vi "Set Values From HovaCAL Output.vi"(8 "error in (no error)":errorcluster caption="Fehler (Eingang, kein Fehler)") -> (0 "error out":errorcluster caption="Fehler (Ausgang)", 1 "Cluster.Flow Output Cluster (Ausgang)":cluster{"total flow":dbl} caption="Flow Output", 2 "Cluster.Pump MassFlow-Cluster":T7(array[cluster]) caption="Pump MassFlow", 3 "Cluster.Pump Concentrations-Cluster":T8(array[cluster]) caption="Pump Output", 4 "Cluster.PumpModeGeneral-Cluster":cluster{"running?":bool, "Speed":dbl[]} caption="Pump Status", 5 "Cluster.Temp Cluster":T1(array[cluster]) caption="Temp Output", 6 "Cluster.MFC Flows-Cluster":T6(array[cluster]), 7 "MFC Input/Output Concentrations (Ausgang)":T9[](array[typedef]) caption="MFC Input/Output" {"Input Concentration" format="%.2f"; "Output Setpoint" format="%.2f"; "flow expected" format="%.2f"; "flow actual" format="%.2f"; "output concentration dry" format="%.2f"; "output concentration" format="%.2f"}, 9 "Water-Cluster out":cluster{"water conc SP":dbl, "water conc":dbl}, 10 "PumpMode-Cluster":T4(array[cluster]) {"concentratio mode" items=["water", "reagent"]; "Reagent" items=["HCl", "HF", "NH3", "HG", "PPM", "ORGANIC"]}, 11 "MFC Output Array":T5[](array[typedef]) {"flow expected" format="%.2f"; "flow actual" format="%.2f"; "output concentration dry" format="%.2f"; "output concentration" format="%.2f"})   [LabVIEW 2020, in "Linearisierung v2.lvlib" / "Gasteiler.lvlib" / "HovaCAL_Interface.lvlib" / "Kommunikation.lvlib"]
uses:
  Kommunikation.lvlib
  Controls/MFC Output.ctl
  Controls/Pump Concentration Mode.ctl
  Controls/Reagent.ctl
  Aktion_FGV_HovaCAL_Interface_GetData.ctl
  Controls/Controls.lvlib
  Controls/MFC Output plus Input Output Concentrations.ctl
panel:
  # "l/min"
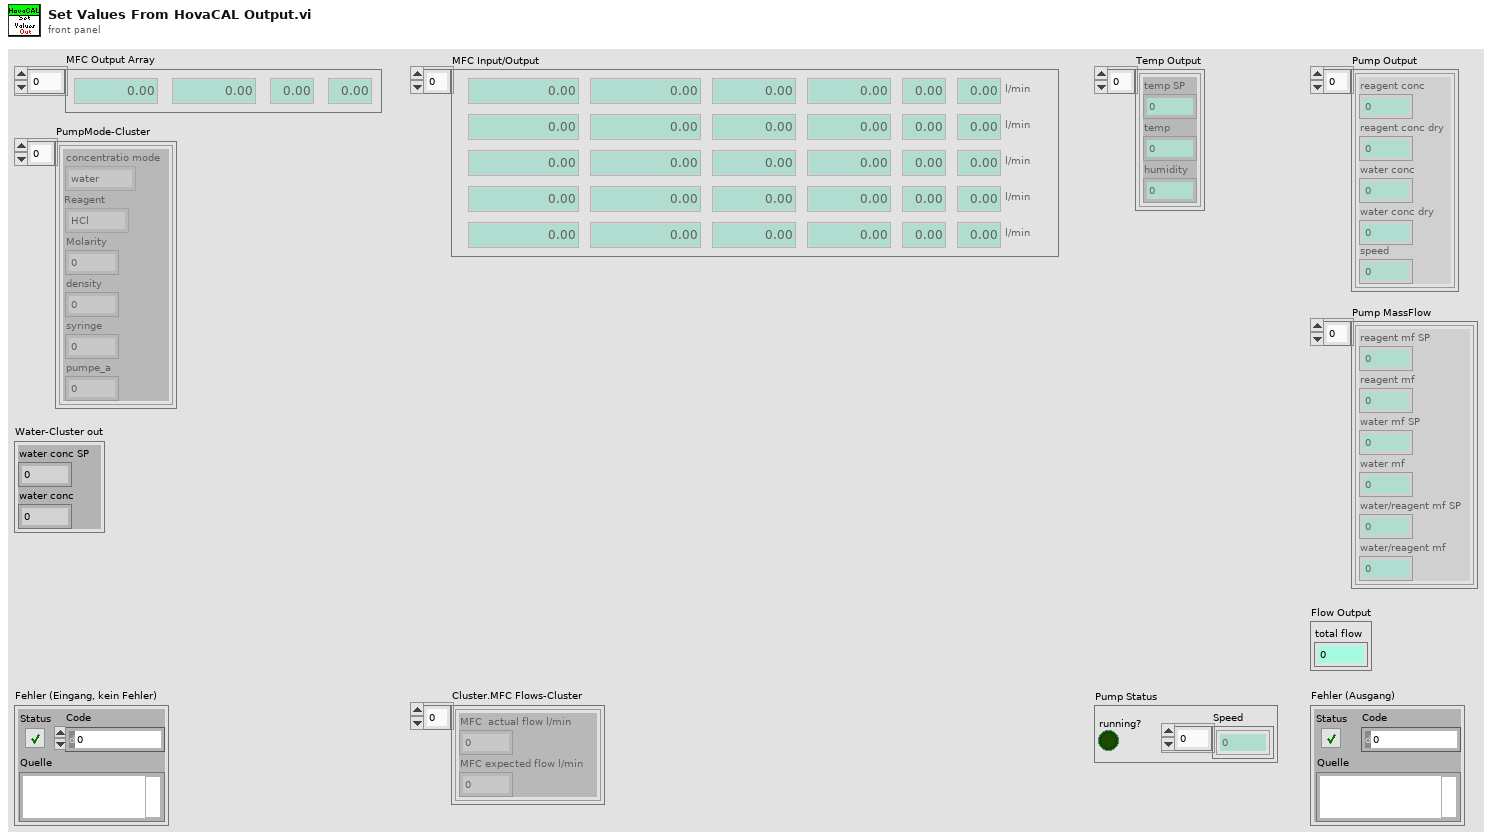
[diagram p1: front panel]
types:
  T1 = cluster{"temp SP":dbl, "temp":dbl, "humidity":dbl}[]
  T2 = typedef "Linearisierung v2.lvlib/Gasteiler.lvlib/HovaCAL_Interface.lvlib/Controls.lvlib/Pump Concentration Mode.ctl" = i32
  T3 = typedef "Linearisierung v2.lvlib/Gasteiler.lvlib/HovaCAL_Interface.lvlib/Controls.lvlib/Reagent.ctl" = i32
  T4 = cluster{"concentratio mode":T2, "Reagent":T3, "Molarity":dbl, "density":dbl, "syringe":dbl, "pumpe_a":dbl}[]
  T5 = typedef "Linearisierung v2.lvlib/Gasteiler.lvlib/HovaCAL_Interface.lvlib/Controls.lvlib/MFC Output.ctl" = cluster{"output concentration":dbl, "output concentration dry":dbl, "flow actual":dbl, "flow expected":dbl}
  T6 = cluster{"MFC  actual flow l/min":dbl, "MFC expected flow l/min":dbl}[]
  T7 = cluster{"reagent mf SP":dbl, "reagent mf":dbl, "water mf SP":dbl, "water mf":dbl, "water/reagent mf SP":dbl, "water/reagent mf":dbl}[]
  T8 = cluster{"reagent conc":dbl, "reagent conc dry":dbl, "water conc":dbl, "water conc dry":dbl, "speed":dbl}[]
  T9 = typedef "Linearisierung v2.lvlib/Gasteiler.lvlib/HovaCAL_Interface.lvlib/Controls.lvlib/MFC Output plus Input Output Concentrations.ctl" = cluster{"Input Concentration":dbl, "Output Setpoint":dbl, "output concentration":dbl, "output concentration dry":dbl, "flow actual":dbl, "flow expected":dbl}
  T10 = cluster{"temp SP":dbl, "temp":dbl, "humidity":dbl}
  T11 = cluster{"concentratio mode":T2, "Reagent":T3, "Molarity":dbl, "density":dbl, "syringe":dbl, "pumpe_a":dbl}
  T12 = cluster{"reagent conc":dbl, "reagent conc dry":dbl, "water conc":dbl, "water conc dry":dbl, "speed":dbl}
  T13 = typedef "Linearisierung v2.lvlib/Gasteiler.lvlib/HovaCAL_Interface.lvlib/Kommunikation.lvlib/Aktion_FGV_HovaCAL_Interface_GetData.ctl" = enum16{"lesen", "SystemInfo", "MFC Info", "actual Values", "Limits", "first contact", "reset after read"}
  T14 = typedef "Linearisierung v2.lvlib/Gasteiler.lvlib/HovaCAL_Interface.lvlib/Controls.lvlib/Pump Dry Mode.ctl" = i32
  T15 = typedef "Linearisierung v2.lvlib/Gasteiler.lvlib/HovaCAL_Interface.lvlib/Controls.lvlib/Pump Control Mode.ctl" = u32
  T16 = cluster{"Input Concentrations (Ausgang)":cluster{"input concentration setpoint":dbl, "output concentration setpoint":dbl, "output concentration":dbl, "output concentration dry":dbl}[], "Cluster":cluster{"Temp Cluster":cluster{"temp SP":dbl, "temp":dbl, "humidity":dbl}[], "PumpModeGeneral-Cluster":cluster{"running?":bool, "dry mode":T14, "control mode":T15}, "PumpMode-Cluster":cluster{"Speed":dbl, "concentratio mode":T2, "Reagent":T3, "Molarity":dbl, "density":dbl, "syringe":dbl, "pumpe_a":dbl}[], "Pump Concentrations-Cluster":cluster{"reagent conc SP":dbl, "reagent conc":dbl, "reagent conc dry":dbl, "water conc SP":dbl, "water conc":dbl, "water conc dry":dbl}[], "Flow Output Cluster (Ausgang)":cluster{"total flow setpoint":dbl, "total flow":dbl}, "Pump MassFlow-Cluster":cluster{"reagent mf SP":dbl, "reagent mf":dbl, "water mf SP":dbl, "water mf":dbl, "water/reagent mf SP":dbl, "water/reagent mf":dbl}[], "MFC Flows-Cluster":cluster{"MFC  actual flow l/min":dbl, "MFC expected flow l/min":dbl}[]}}
  T17 = cluster{"input concentration setpoint":dbl, "output concentration setpoint":dbl, "output concentration":dbl, "output concentration dry":dbl}[]
  T18 = cluster{"running?":bool, "dry mode":T14, "control mode":T15}
  T19 = cluster{"Speed":dbl, "concentratio mode":T2, "Reagent":T3, "Molarity":dbl, "density":dbl, "syringe":dbl, "pumpe_a":dbl}[]
  T20 = cluster{"reagent conc SP":dbl, "reagent conc":dbl, "reagent conc dry":dbl, "water conc SP":dbl, "water conc":dbl, "water conc dry":dbl}[]
  T21 = cluster{"total flow setpoint":dbl, "total flow":dbl}
  T22 = cluster{"reagent conc SP":dbl, "reagent conc":dbl, "reagent conc dry":dbl, "water conc SP":dbl, "water conc":dbl, "water conc dry":dbl}
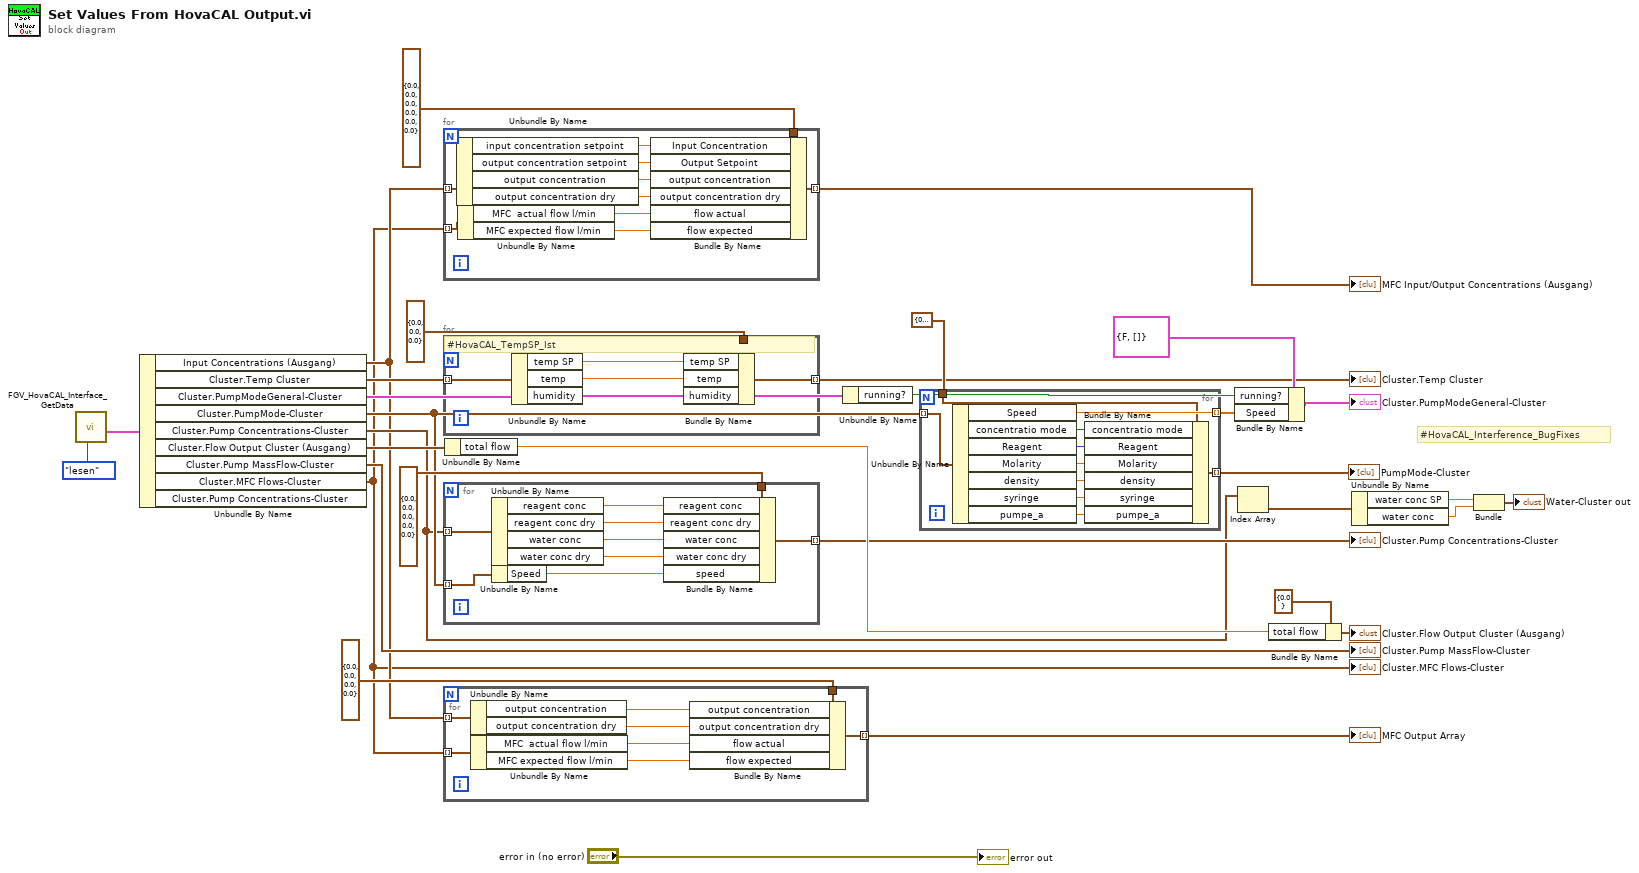
[diagram p0: block diagram]
diagram:
  # "#HovaCAL_Interference_BugFixes"
  n1 = call "FGV_HovaCAL_Interface_GetData.vi"("Aktion"=Aktion_FGV_HovaCAL_Interface_GetData."lesen") -> ("actual Values Cluster out"=w31:T16)  [unwired: 6 in, 4 out]
  n2 = Unbundle By Name(w31) -> ("Input Concentrations (Ausgang)"=w4:T17, "Cluster.Temp Cluster"=w30:T1, "Cluster.PumpModeGeneral-Cluster"=w28:T18, "Cluster.PumpMode-Cluster"=w9:T19, "Cluster.Pump Concentrations-Cluster"=w6:T20, "Cluster.Flow Output Cluster (Ausgang)"=w23:T21, "Cluster.Pump MassFlow-Cluster"=→"Cluster.Pump MassFlow-Cluster":T7, "Cluster.MFC Flows-Cluster"=w2:T6)  [unwired: 1 out]
  "Cluster.MFC Flows-Cluster" <- w2
  n3 = for {
    tunnel: w4 -> [w41] mode=indexing
    tunnel: T9 {"Input Concentration"=0.0, "Output Setpoint"=0.0, "output concentration"=0.0, "output concentration dry"=0.0, "flow actual"=0.0, "flow expected"=0.0} ("Actual Values Cluster") -> [w42]
    tunnel: [w39] -> w1 mode=indexing
    tunnel: w2 -> [w37] mode=indexing
    n4 = Unbundle By Name(w41) -> ("input concentration setpoint"=w33:dbl, "output concentration setpoint"=w34:dbl, "output concentration"=w40:dbl, "output concentration dry"=w38:dbl)
    n5 = Unbundle By Name(w37) -> ("MFC  actual flow l/min"=w35:dbl, "MFC expected flow l/min"=w36:dbl)
    n6 = Bundle By Name(cluster=w42, "Input Concentration"=w33, "Output Setpoint"=w34, "output concentration"=w40, "output concentration dry"=w38, "flow actual"=w35, "flow expected"=w36) -> (w39:T9)
  }
  "MFC Input/Output Concentrations (Ausgang)" <- w1
  n7 = for {
    tunnel: w30 -> [w48] mode=indexing
    tunnel: [w46] -> w13 mode=indexing
    tunnel: T10 {"temp SP"=0.0, "temp"=0.0, "humidity"=0.0} ("Temp Cluster") -> [w44]
    # "#HovaCAL_TempSP_Ist"
    n8 = Unbundle By Name(w48) -> ("temp SP"=w43:dbl, "temp"=w47:dbl, "humidity"=w45:dbl)
    n9 = Bundle By Name(cluster=w44, "temp SP"=w43, "temp"=w47, "humidity"=w45) -> (w46:T10)
  }
  "Cluster.Temp Cluster" <- w13
  n10 = for {
    tunnel: w6 -> [w56] mode=indexing
    tunnel: T12 {"reagent conc"=0.0, "reagent conc dry"=0.0, "water conc"=0.0, "water conc dry"=0.0, "speed"=0.0} ("Ausgangs-Cluster") -> [w57]
    tunnel: [w54] -> w11 mode=indexing
    tunnel: w9 -> [w50] mode=indexing
    n11 = Unbundle By Name(w56) -> ("reagent conc"=w55:dbl, "reagent conc dry"=w53:dbl, "water conc"=w52:dbl, "water conc dry"=w51:dbl)
    n12 = Unbundle By Name(w50) -> ("Speed"=w49:dbl)
    n13 = Bundle By Name(cluster=w57, "reagent conc"=w55, "reagent conc dry"=w53, "water conc"=w52, "water conc dry"=w51, "speed"=w49) -> (w54:T12)
  }
  "Cluster.Pump Concentrations-Cluster" <- w11
  n14 = for {
    tunnel: w2 -> [w64] mode=indexing
    tunnel: T5 {"output concentration"=0.0, "output concentration dry"=0.0, "flow actual"=0.0, "flow expected"=0.0} ("MFC Output") -> [w65]
    tunnel: [w63] -> w18 mode=indexing
    tunnel: w4 -> [w58] mode=indexing
    n15 = Unbundle By Name(w58) -> ("output concentration"=w60:dbl, "output concentration dry"=w59:dbl)
    n16 = Unbundle By Name(w64) -> ("MFC  actual flow l/min"=w62:dbl, "MFC expected flow l/min"=w61:dbl)
    n17 = Bundle By Name(cluster=w65, "output concentration"=w60, "output concentration dry"=w59, "flow actual"=w62, "flow expected"=w61) -> (w63:T5)
  }
  "MFC Output Array" <- w18
  n18 = Unbundle By Name(w23) -> ("total flow"=w21:dbl)
  n19 = Unbundle By Name(w28) -> ("running?"=w27:bool)
  n20 = for {
    tunnel: w9 -> [w75] mode=indexing
    tunnel: [w74] -> w25 mode=indexing
    tunnel: T11 {"concentratio mode"=0, "Reagent"=0, "Molarity"=0.0, "density"=0.0, "syringe"=0.0, "pumpe_a"=0.0} ("PumpMode-Cluster") -> [w73]
    tunnel: [w66] -> w12 mode=indexing
    n21 = Unbundle By Name(w75) -> ("Speed"=w74:dbl, "concentratio mode"=w72:T2, "Reagent"=w71:T3, "Molarity"=w70:dbl, "density"=w69:dbl, "syringe"=w68:dbl, "pumpe_a"=w67:dbl)
    n22 = Bundle By Name(cluster=w73, "concentratio mode"=w72, "Reagent"=w71, "Molarity"=w70, "density"=w69, "syringe"=w68, "pumpe_a"=w67) -> (w66:T11)
  }
  "PumpMode-Cluster" <- w12
  n23 = Bundle By Name(cluster=cluster{"running?":bool, "Speed":dbl[]} {"running?"=FALSE, "Speed"=[]} ("Cluster.PumpModeGeneral-Cluster"), "running?"=w27, "Speed"=w25) -> (→"Cluster.PumpModeGeneral-Cluster":cluster{"running?":bool, "Speed":dbl[]})
  n24 = Index Array(array=w6) -> (element=w5:T22)  [unwired: 1 in]
  n25 = Bundle By Name(cluster=cluster{"total flow":dbl} {"total flow"=0.0} ("Cluster.Flow Output Cluster (Ausgang)"), "total flow"=w21) -> (→"Cluster.Flow Output Cluster (Ausgang)":cluster{"total flow":dbl})
  n26 = Unbundle By Name(w5) -> ("water conc SP"=w10:dbl, "water conc"=w8:dbl)
  n27 = Bundle("water conc SP"=w10, "water conc"=w8) -> (→"Water-Cluster out":cluster{"water conc SP":dbl, "water conc":dbl})  [unwired: 1 in]
  "error out" <- "error in (no error)"
